vi "sample-profiled-pid-linear.vi"() -> ()   [LabVIEW 2019]
uses:
  <vilib>/Rock Robotics/WPI/ThirdParty/JAS_Junk/TrajLib/TrapProfState_New.vi
  <vilib>/Rock Robotics/WPI/ThirdParty/JAS_Junk/TrajLib/PIDController_NewPeriod.vi
  <vilib>/Rock Robotics/SystemInterfaces/NetworkCommunication/NetComm_UsageReport_report.vi
  <vilib>/Rock Robotics/WPI/ThirdParty/JAS_Junk/TrajLib/PIDController_SetIntegratorRange.vi
  <vilib>/Rock Robotics/WPI/ThirdParty/JAS_Junk/TrajLib/PIDController_SetTolerancePandV.vi
  <vilib>/Rock Robotics/WPI/ThirdParty/JAS_Junk/TrajLib/ProfiledPIDController_Reset.vi
  <vilib>/Rock Robotics/WPI/ThirdParty/JAS_Junk/TrajLib/LinearFilter_ResetToValue.vi
  <vilib>/Rock Robotics/WPI/ThirdParty/JAS_Junk/TrajLib/LinearFilter_Calculate.vi
  <vilib>/Rock Robotics/WPI/ThirdParty/JAS_Junk/TrajLib/ProfiledPIDController_SetGoal_PosOnly.vi
  <vilib>/Rock Robotics/WPI/ThirdParty/JAS_Junk/TrajLib/ProfiledPIDController_Calculate_Meas.vi
  <vilib>/Rock Robotics/WPI/ThirdParty/JAS_Junk/TrajLib/PIDController_GetVelocityError.vi
  <vilib>/Rock Robotics/WPI/ThirdParty/JAS_Junk/TrajLib/PIDController_GetPositionError.vi
  <vilib>/Rock Robotics/WPI/ThirdParty/JAS_Junk/TrajLib/PIDController_AtSetpoint.vi
  <vilib>/Rock Robotics/WPI/ThirdParty/JAS_Junk/TrajLib/TrapProfState_Equals.vi
  <vilib>/Rock Robotics/WPI/ThirdParty/JAS_Junk/TrajLib/PIDController_Reset.vi
  <vilib>/Rock Robotics/WPI/ThirdParty/JAS_Junk/TrajLib/ProfiledPIDController_SetGoal.vi
  <vilib>/Rock Robotics/WPI/ThirdParty/JAS_Junk/TrajLib/PIDController_Calculate_SP_PV.vi
  <vilib>/Rock Robotics/WPI/ThirdParty/JAS_Junk/TrajLib/TrapProfile_New.vi
  <vilib>/Rock Robotics/WPI/ThirdParty/JAS_Junk/TrajLib/ProfiledPIDController_GetPeriod.vi
  <vilib>/Rock Robotics/WPI/ThirdParty/JAS_Junk/TrajLib/TrapProfile_Calculate.vi
  <vilib>/Rock Robotics/WPI/ThirdParty/JAS_Junk/TrajLib/ControllerUtil_GetModulusError.vi
  <vilib>/Rock Robotics/WPI/ThirdParty/JAS_Junk/TrajLib/PIDController_SetSetpoint.vi
  <vilib>/Rock Robotics/WPI/ThirdParty/JAS_Junk/TrajLib/PIDController_Calculate_PV.vi
  <vilib>/Rock Robotics/WPI/ThirdParty/JAS_Junk/TrajLib/TrapProfile_ShouldFlipAcceleration.vi
  <vilib>/Rock Robotics/WPI/ThirdParty/JAS_Junk/TrajLib/TrapProfile_Direct.vi
  <vilib>/Rock Robotics/WPI/ThirdParty/JAS_Junk/TrajLib/PIDController_GetPeriod.vi
  <vilib>/Rock Robotics/WPI/ThirdParty/JAS_Junk/TrajLib/Util_LibraryGlobals.vi
  <vilib>/Rock Robotics/WPI/ThirdParty/JAS_Junk/TrajLib/LinearFilter_MovingAverage.vi
  <vilib>/Rock Robotics/WPI/ThirdParty/JAS_Junk/TrajLib/LinearFilter_LowPassBW1.vi
  <vilib>/Rock Robotics/WPI/ThirdParty/JAS_Junk/TrajLib/LinearFilter_LowPassBW2.vi
  <vilib>/Rock Robotics/WPI/ThirdParty/JAS_Junk/TrajLib/LinearFilter_HighPassBW1.vi
  <vilib>/Rock Robotics/WPI/ThirdParty/JAS_Junk/TrajLib/LinearFilter_HighPassBW2.vi
  <vilib>/Rock Robotics/WPI/ThirdParty/JAS_Junk/TrajLib/Trajectory_Library.lvlib
  <vilib>/ptbypt/NI_PtbyPt.lvlib
panel:
  in  "Tab Control":enum32{"Operation", "Tuning"}(tab)
  out "Targets along the way":T1(graph)
  in  "SP - Desired Position\n (Inch)":dbl(slide) scale=-10.0..350.0
  out "PV - Current Position\n (Inch)":dbl(slide) scale=-10.0..350.0
  out "Goal":T2(graph)
  out "Motor Output":dbl format="%13.3f"
  out "AtSetpoint":bool
  out "AtGoal":bool
  out "PositionError  (Inch)":dbl format="%13.2f"
  out "VelocityError  (Inch/Sec)":dbl format="%13.2f"
  out "Velocity  (Inch/Sec)":dbl format="%13.2f"
  in  "Kp":dbl=0.08 format="%#_13g"
  in  "Ki":dbl=0.15 format="%#_13g"
  in  "Kd":dbl format="%#_13g"
  in  "Minimum Integral":dbl=-0.3 format="%#_13g"
  in  "Maximum Integral":dbl=0.3 format="%#_13g"
  in  "Max Speed   (Inch/Sec)":dbl=30.0 format="%#_13g"
  in  "Max Accel  (Inch/Sec^2)":dbl=5.0 format="%#_13g"
  in  "PositionTolerance\n(Inch)":dbl=1.0 format="%#_13g"
  in  "VelocityTolerance\n(Inch/Sec)":dbl=0.05 format="%#_13g"
  # "Position has hard limit\n at -5 and 300 inches"
  # "SET THESE BEFORE EXECUTING THIS PROGRAM."
  # "PID Tuning Parameters"
  # "Desired Profile Performance"
  # "Desired On Target Tolerance"
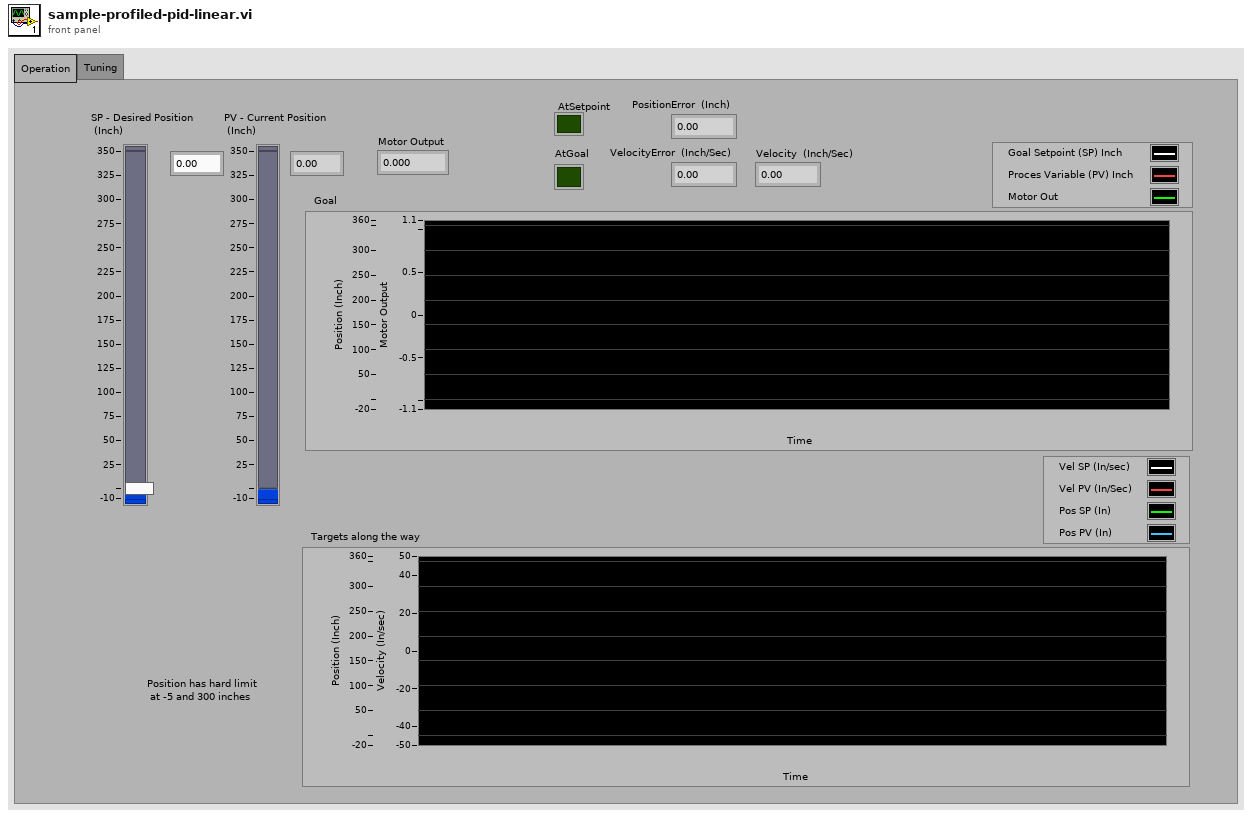
[diagram p1: front panel]
types:
  T1 = cluster{"SP - Desired Heading\n (Deg)":dbl, "PV - Current Heading\n (Deg)":dbl, "upper limit":dbl, dbl}
  T2 = cluster{"SP - Desired Position\n (Inch)":dbl, "upper limit":dbl, "upper limit":dbl}
  T3 = typedef "Trajectory_Library.lvlib/TRAPEZOID_PROFILE_CONSTRAINT.ctl" = cluster{"MaxVelocity":dbl, "MaxAcceleration":dbl}
  T4 = typedef "Trajectory_Library.lvlib/PROFILED_PID_CONTROLLER.ctl" = cluster{"Controller":T5, "Goal":T6, "Setpoint":T6, "Constraint":T3}
  T5 = typedef "Trajectory_Library.lvlib/PID_CONTROLLER.ctl" = cluster{"Kp":dbl, "Ki":dbl, "Kd":dbl, "Period":dbl, "Max_Integral":dbl, "Min_Integral":dbl, "Max_Input":dbl, "Min_Input":dbl, "Continuous":bool, "PositionError":dbl, "VelocityError":dbl, "PrevError":dbl, "TotalError":dbl, "PositionTolerance":dbl, "VelocityTolerance":dbl, "SetPoint":dbl, "Kf":dbl, "Prev_Deriv":dbl, "Prev_Deriv 2":dbl, "DerivativeFilter":bool, "Min_Output":dbl, "Max_Output":dbl, "Prev_F_P":dbl, "Prev_F_P_2":dbl, "AntiWindupActive":bool, "Measurement":dbl}
  T6 = typedef "Trajectory_Library.lvlib/TRAPEZOID_PROFILE_STATE.ctl" = cluster{"Position":dbl, "Velocity":dbl}
  T7 = enum16{"Moving Average", "Low Pass 1st Order Butterworth", "Low Pass 2nd Order Butterworth", "High Pass 1st Order Butterworth", "High Pass 2nd Order Butterworth"}
  T8 = cluster{"Velocity":dbl, dbl, "Position":dbl, "upper limit":dbl}
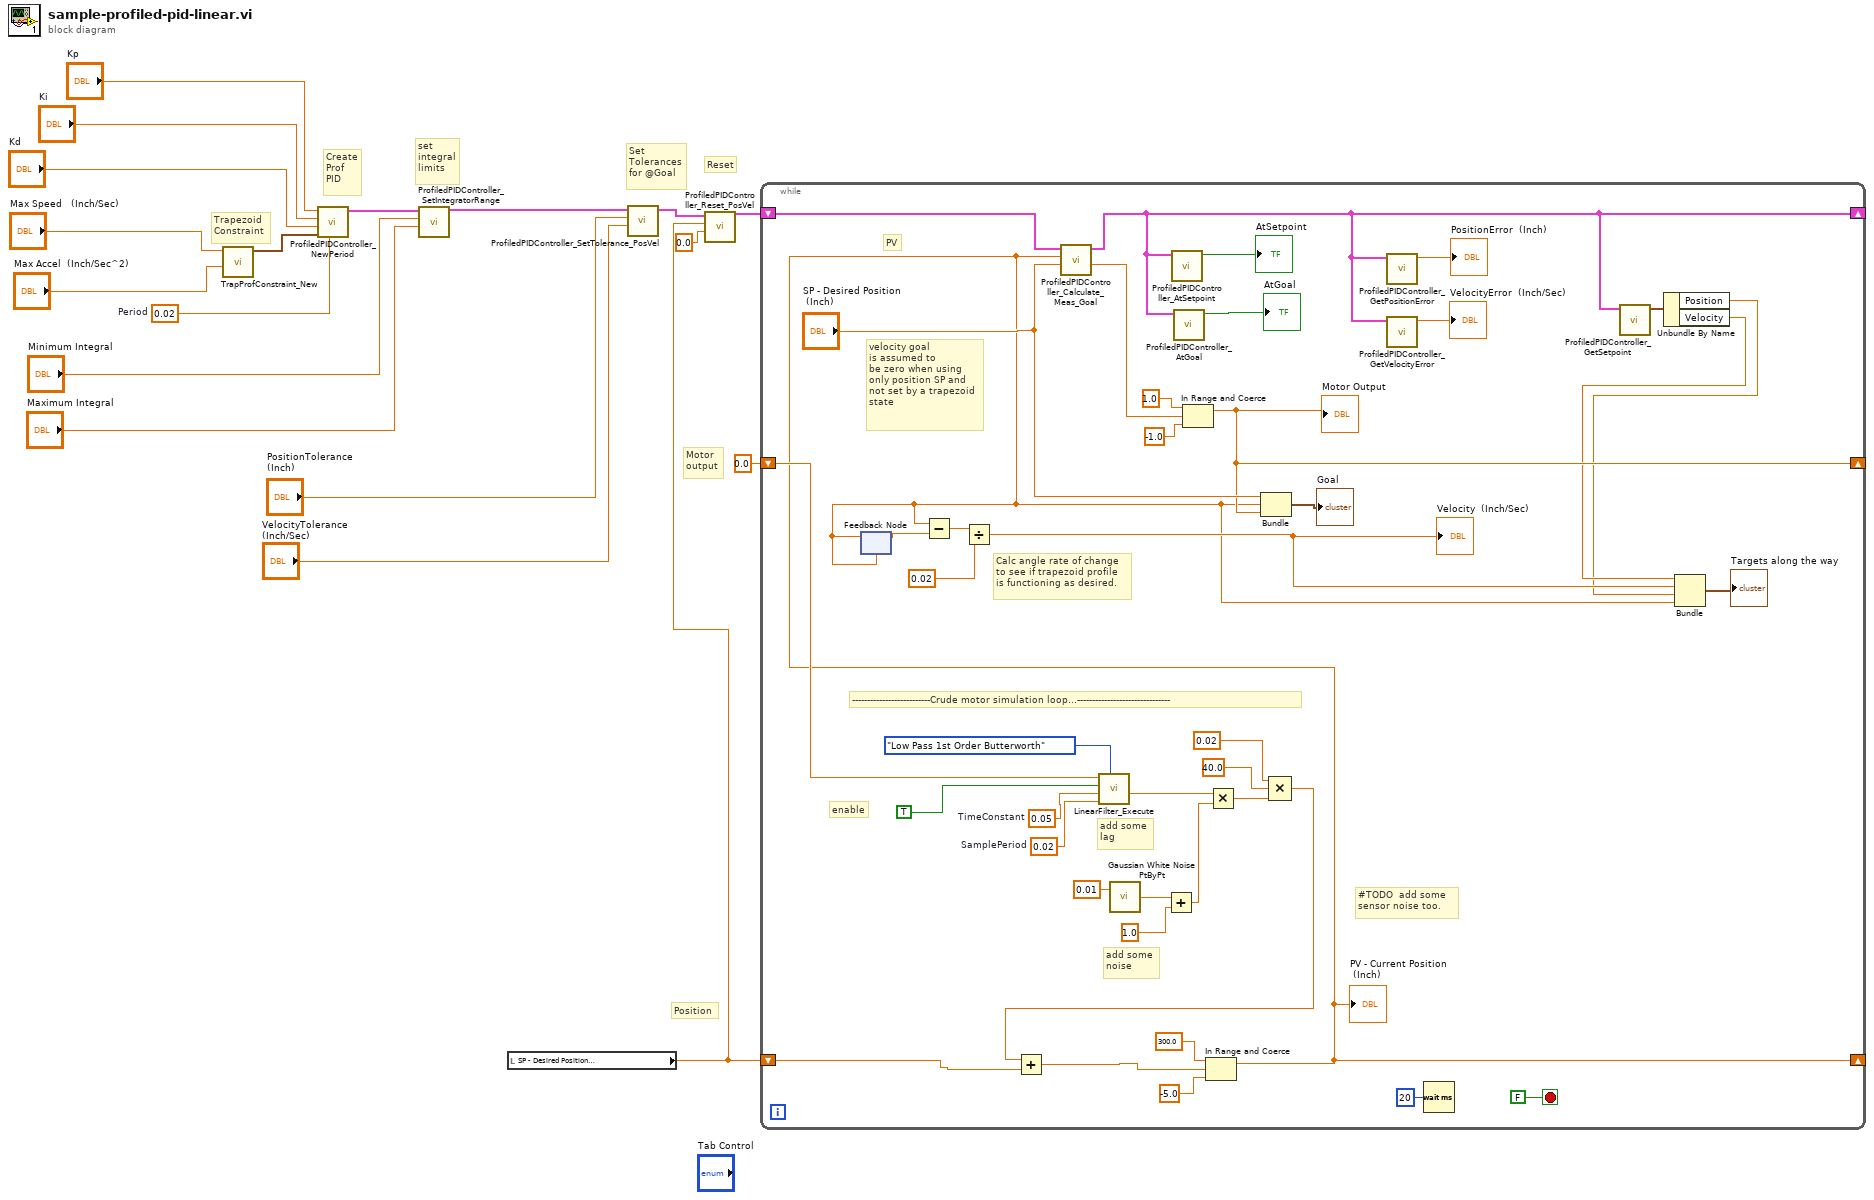
[diagram p0: block diagram]
diagram:
  w15 = 0.02  # Period
  # "Reset"
  # "Position"
  # "Motor\noutput"
  # "set\nintegral\nlimits"
  # "Trapezoid\nConstraint"
  # "Set\nTolerances\nfor @Goal"
  # "Create\nProf\nPID"
  n1 = call <vilib>:"TrapProfConstraint_New.vi"("Max Accel"="Max Accel  (Inch/Sec^2)", "Max Speed (M/S)"="Max Speed   (Inch/Sec)") -> ("TRAPEZOID_PROFILE_CONSTRAINT"=w18:T3)  [unwired: 9 in]
  n2 = call <vilib>:"ProfiledPIDController_NewPeriod.vi"("Period"=w15, "Constraints"=w18, "Kd"="Kd", "Ki"="Ki", "Kp"="Kp") -> ("PROFILED_PID_CONTROLLER"=w9:T4)  [unwired: 6 in]
  n3 = call <vilib>:"ProfiledPIDController_SetIntegratorRange.vi"("Maximum"="Maximum Integral", "Minimum"="Minimum Integral", "in PROFILED_PID_CONTROLLER"=w9) -> ("out PROFILED_PID_CONTROLLER"=w1:T4)  [unwired: 8 in]
  n4 = local read "SP - Desired Position\n (Inch)"() -> (w2:dbl)
  n5 = call <vilib>:"ProfiledPIDController_SetTolerance_PosVel.vi"("VelocityTolerance"="VelocityTolerance\n(Inch/Sec)", "PositionTolerance"="PositionTolerance\n(Inch)", "in PROFILED_PID_CONTROLLER"=w1) -> ("out PROFILED_PID_CONTROLLER"=w4:T4)  [unwired: 8 in]
  n6 = call <vilib>:"ProfiledPIDController_Reset_PosVel.vi"("Velocity"=0.0, "Position"=w2, "in PROFILED_PID_CONTROLLER"=w4) -> ("out PROFILED_PID_CONTROLLER"=w5:T4)  [unwired: 8 in]
  n7 = while {
    shift-right: [w24] -> _
    shift-left: w5 -> [w59]
    shift-right: [w19] -> _
    shift-left: w2 -> [w32]
    shift-right: [w31] -> _
    shift-left: 0.0 ("upper limit") -> [w30]
    stop <- FALSE stop-if-true
    w34 = 0.02  # SamplePeriod
    w33 = 0.05  # TimeConstant
    # "enable"
    # "PV"
    # "#TODO  add some\nsensor noise too."
    # "add some\nnoise"
    # "add some\nlag"
    # "--------------------------Crude motor simulation loop...-------------------------------"
    # "Calc angle rate of change\nto see if trapezoid profile\nis functioning as desired."
    # "velocity goal\nis assumed to \nbe zero when using\nonly position SP and\nnot set by a trapezoid\nstate"
    n8 = call <vilib>:"LinearFilter_Execute.vi"("Filter Type"=T7."Low Pass 1st Order Butterworth", "SamplePeriod"=w34, "TimeConstant"=w33, "Enable"=TRUE, "Input"=w30) -> ("Output"=w41:dbl)  [unwired: 5 in, 1 out]
    n9 = call <vilib>:"Gaussian White Noise PtByPt.vi"("standard deviation"=0.01) -> ("Gaussian white noise"=w40:dbl)  [unwired: 2 in]
    n10 = Add(x=w40, y=1.0) -> (x+y=w42:dbl)
    n11 = Multiply(x=w41, y=w42) -> (x*y=w43:dbl)
    n12 = Compound Arithmetic op=MULTIPLY(0.02 ("value"), 40.0 ("value"), w43) -> (w44:dbl)
    n13 = Add(x=w44, y=w32) -> (x+y=w28:dbl)
    n14 = In Range and Coerce(upper limit=300.0, x=w28, lower limit=-5.0) -> (coerced(x)=w19:dbl)  [unwired: 1 out]
    "PV - Current Position\n (Inch)" <- w19
    n15 = feedback-in #1(w19) -> ()
    n16 = feedback #1(w19) -> (w51:dbl)
    n17 = Subtract(x=w19, y=w51) -> (x-y=w50:dbl)
    n18 = Divide(x=w50, y=0.02) -> (x/y=w21:dbl)
    "Velocity  (Inch/Sec)" <- w21
    n19 = call <vilib>:"ProfiledPIDController_Calculate_Meas_Goal.vi"("SP-Goal"="SP - Desired Position\n (Inch)", "PV-Measurement"=w19, "in PROFILED_PID_CONTROLLER"=w59) -> ("CO-ControlOutput"=w52:dbl, "out PROFILED_PID_CONTROLLER"=w24:T4)  [unwired: 7 in]
    n20 = call <vilib>:"ProfiledPIDController_AtSetpoint.vi"("in PROFILED_PID_CONTROLLER"=w24) -> ("AtSetpoint"=→"AtSetpoint":bool)  [unwired: 10 in]
    n21 = call <vilib>:"ProfiledPIDController_AtGoal.vi"("in PROFILED_PID_CONTROLLER"=w24) -> ("AtGoal"=→"AtGoal":bool)  [unwired: 10 in]
    n22 = In Range and Coerce(upper limit=1.0, x=w52, lower limit=-1.0) -> (coerced(x)=w31:dbl)  [unwired: 1 out]
    "Motor Output" <- w31
    n23 = Bundle("SP - Desired Position\n (Inch)"="SP - Desired Position\n (Inch)", "upper limit"=w19, "upper limit"=w31) -> (→"Goal":T2)  [unwired: 1 in]
    n24 = call <vilib>:"ProfiledPIDController_GetPositionError.vi"("in PROFILED_PID_CONTROLLER"=w24) -> ("PositionError"=→"PositionError  (Inch)":dbl)  [unwired: 10 in]
    n25 = call <vilib>:"ProfiledPIDController_GetVelocityError.vi"("in PROFILED_PID_CONTROLLER"=w24) -> ("VelocityError"=→"VelocityError  (Inch/Sec)":dbl)  [unwired: 10 in]
    n26 = Wait (ms)(milliseconds to wait=u32 20) -> ()  [unwired: 1 out]
    n27 = call <vilib>:"ProfiledPIDController_GetSetpoint.vi"("in PROFILED_PID_CONTROLLER"=w24) -> ("Setpoint"=w23:T6)  [unwired: 10 in]
    n28 = Unbundle By Name(w23) -> ("Position"=w20:dbl, "Velocity"=w22:dbl)
    n29 = Bundle("Velocity"=w22, w21, "Position"=w20, "upper limit"=w19) -> (→"Targets along the way":T8)  [unwired: 1 in]
  }
